vi "Run Child.vi"(8 "error in (no error)":errorcluster, 9 "Working Path":path, 10 "UI":refnum<class "UI.lvclass">, 11 "Help in":refnum<class "Help.lvclass">) -> (0 "error out":errorcluster, 3 "Help out":refnum<class "Help.lvclass">)   [LabVIEW 2020, in "Help.lvlib" / "Help.lvclass"]
uses:
  Help.lvclass
  build/ppl/neg-pkg.lvlibp/neg-pkg/UI/UI.lvclass
  Help.lvclass/Help.ctl
  build/ppl/neg-pkg.lvlibp/neg-pkg/Action/Action.lvclass
  build/ppl/neg-pkg.lvlibp/neg-pkg/Plugin/Plugin.lvclass
  C:/dev/LabVIEW/build/ppl/neg-pkg.lvlibp/neg-pkg/Plugin/Plugin.lvclass
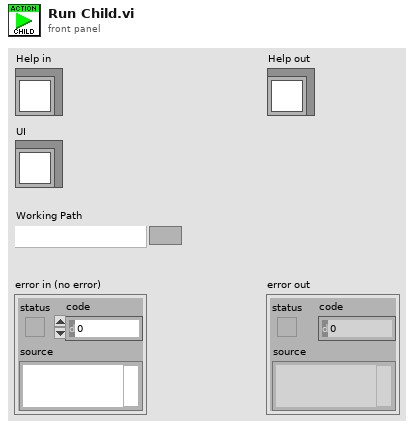
[diagram p1: front panel]
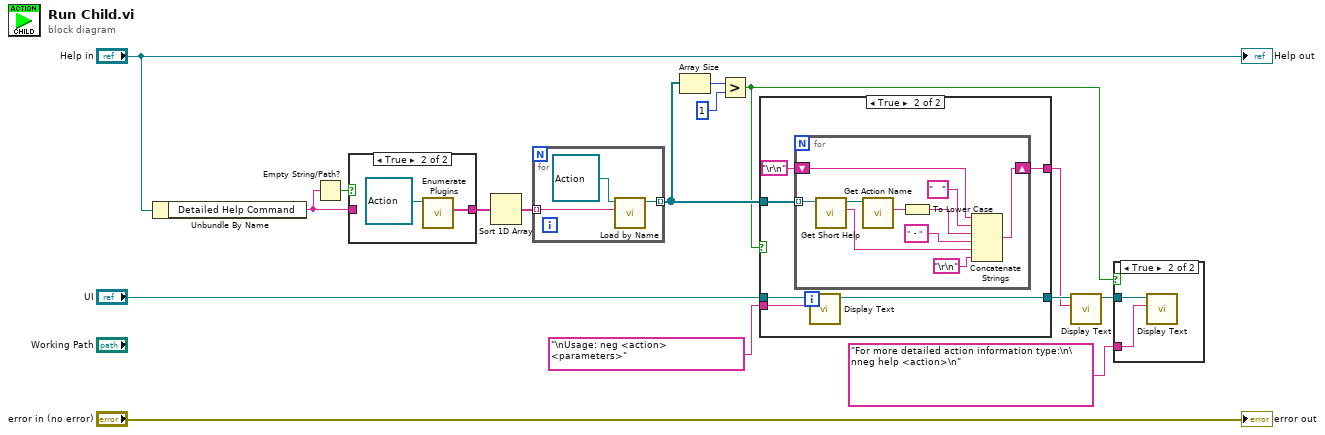
[diagram p0: block diagram]
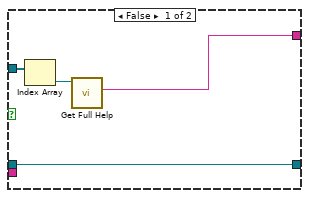
[diagram p3: hidden frame]
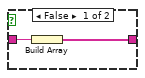
[diagram p4: hidden frame]
diagram:
  n1 = Unbundle By Name("Help in") -> ("Detailed Help Command"=w14:string)
  n2 = Empty String/Path?(string/path=w14) -> (empty?=w15:bool)
  n3 = case shown="True" w15 {
    tunnel: [w17 w19] -> w13
    tunnel: w14 -> [w18 _]
    frame False {
      n4 = Build Array(w18) -> (w17:string[])
    }
    frame True {
      n5 = call "Enumerate Plugins.vi"("Plugin in"=refnum<class "Action.lvclass"> refnum ("neg-pkg.lvlibp:Action.lvclass")) -> ("Available Plugins"=w19:string[])  [unwired: 8 in, 2 out]
    }
  }
  n6 = Sort 1D Array(array=w13) -> (sorted array=w12:string[])
  n7 = for {
    tunnel: w12 -> [w23] mode=indexing
    tunnel: [w21] -> w9 mode=indexing
    n8 = call "Load by Name.vi"("Name"=w23, "Plugin in"=refnum<class "Action.lvclass"> refnum ("neg-pkg.lvlibp:Action.lvclass")) -> ("Plugin out"=w21:refnum<class "Action.lvclass">)  [unwired: 8 in, 1 out]
  }
  n9 = Array Size(array=w9) -> (size(s)=w11:i32)
  n10 = Greater?(x=w11, y=1) -> (0:w5:bool)
  n11 = case shown="True" w5 {
    tunnel: w9 -> [w27 w33]
    tunnel: [w24 w32] -> w3
    tunnel: "\nUsage: neg <action> <parameters>" ("Message") -> [_ w31]
    tunnel: "UI" -> [w26 w30]
    tunnel: [w26 w29] -> w4
    frame False {
      n12 = Index Array(array=w27) -> (element=w25:refnum<class "Action.lvclass">)  [unwired: 1 in]
      n13 = call-dynamic "Get Full Help.vi"("Action in"=w25) -> ("Full Help"=w24:string)  [unwired: 8 in, 2 out]
    }
    frame True {
      n14 = for {
        tunnel: w33 -> [w43] mode=indexing
        shift-right: [w35] -> w32
        shift-left: "\r\n" -> [w36]
        n15 = call-dynamic "Get Short Help.vi"("Action in"=w43) -> ("Short Help"=w38:string, "Action out"=w42:refnum<class "Action.lvclass">)  [unwired: 8 in, 1 out]
        n16 = call "Get Action Name.vi"("Action in"=w42) -> ("Action Name"=w41:string)  [unwired: 8 in, 2 out]
        n17 = To Lower Case(string=w41) -> (all lower case string=w40:string)
        n18 = Concatenate Strings(w36, "   " ("string"), w40, "  - " ("string"), w38, "\r\n") -> (w35:string)
      }
      n19 = call-dynamic "Display Text.vi"("Text"=w31, "UI in"=w30) -> ("UI out"=w29:refnum<class "UI.lvclass">)  [unwired: 8 in, 1 out]
    }
  }
  n20 = call-dynamic "Display Text.vi"("Text"=w3, "UI in"=w4) -> ("UI out"=w2:refnum<class "UI.lvclass">)  [unwired: 8 in, 1 out]
  n21 = case shown="True" w5 {
    tunnel: w2 -> [_ w45]
    tunnel: "For more detailed action information type:\n\nneg help <action>\n" ("Message") -> [_ w44]
    frame False {
    }
    frame True {
      n22 = call-dynamic "Display Text.vi"("Text"=w44, "UI in"=w45) -> ()  [unwired: 8 in, 2 out]
    }
  }
  "error out" <- "error in (no error)"
  "Help out" <- "Help in"
